vi "ziListNodesJSON.vi"(0 "Handle In":T2 {"Handle" format="0x%08x"; "Conn" format="0x%08x"}, 5 "Path (\"\")":string, 9 "Flags (None)":T3, 11 "Error In":errorcluster) -> (4 "Handle Out":T2 {"Handle" format="0x%08x"; "Conn" format="0x%08x"}, 6 "Doc":T1(array[cluster]), 15 "Error Out":errorcluster)   [LabVIEW 2018, in "Zurich Instruments LabOne.lvlib"]
doc: "Returns <b> nodes documentation </b> found at the specified path. The path may contain wild cards so that the rertuned nodes do not necessarily have to have the same parents."
uses:
  Zurich Instruments LabOne.lvlib
  <instrlib>/Zurich Instruments LabOne/Private/ziLV64.framework
  <vilib>/regexp/Match Regular Expression.xnode
  ziTypeHandle.ctl
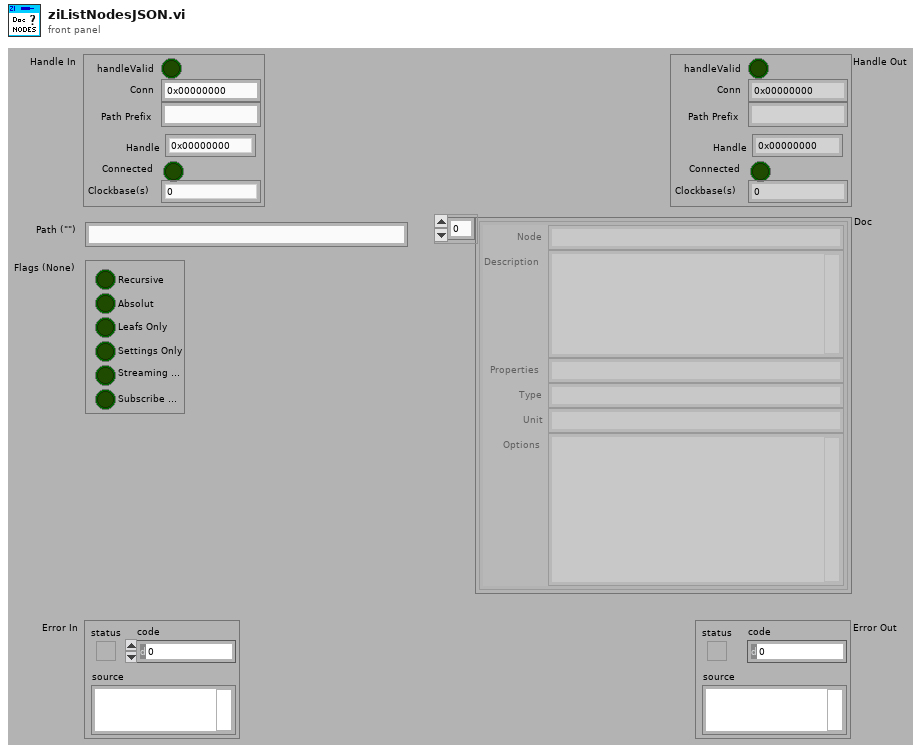
[diagram p1: front panel]
types:
  T1 = cluster{"Node":string, "Description":string, "Properties":string, "Type":string, "Unit":string, "Options":string}[]
  T2 = typedef "Zurich Instruments LabOne.lvlib/ziTypeHandle.ctl" = cluster{"handleValid":bool, "Conn":u64, "Path Prefix":string, "Handle":u64, "Connected":bool, "Clockbase(s)":dbl}
  T3 = cluster{"Recursive":bool, "Absolut":bool, "Leafs Only":bool, "Settings Only":bool, "Streaming Only":bool, "Subscribe Only":bool}
  T4 = cluster{"Node":string, "Description":string, "Properties":string, "Type":string, "Unit":string, "Options":string}
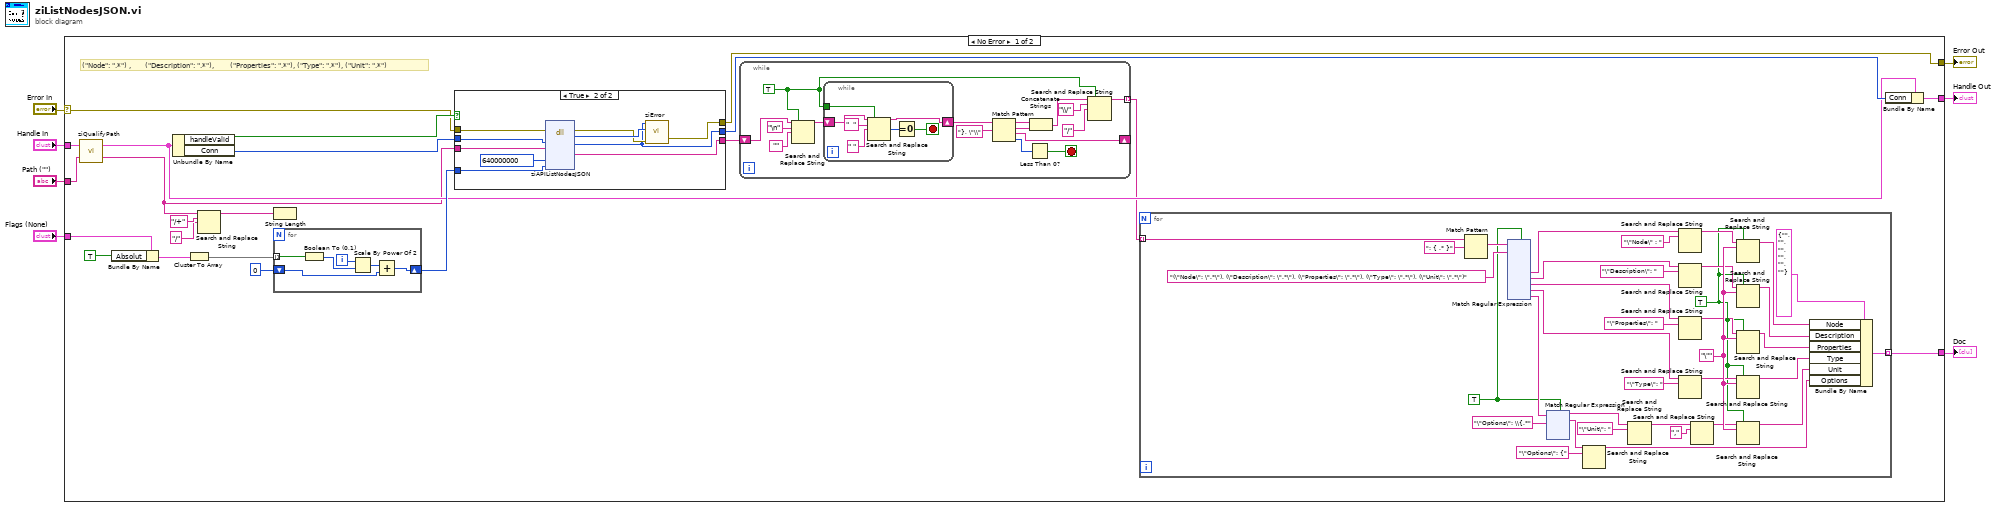
[diagram p0: block diagram]
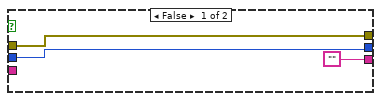
[diagram p2: hidden frame]
diagram:
  n1 = case shown="No Error" "Error In" {
    selector: "Error In" -> [w11 w329]
    tunnel: [w29 w329] -> w7
    tunnel: [w22 w328] -> w6
    tunnel: "Path (\"\")" -> [w21 _]
    tunnel: "Handle In" -> [w20 w328]
    tunnel: "Flags (None)" -> [w17 _]
    tunnel: [w9 _] -> w1
    frame No Error {
      # "(\"Node\": \".*\") ,       (\"Description\": \".*\"),        (\"Properties\": \".*\"), (\"Type\": \".*\"), (\"Unit\": \".*\")"
      n2 = call "ziQualifyPath.vi"("Path In"=w21, "Handle In"=w20) -> ("Path Out"=w12:string, "Handle Out"=w19:T2)
      n3 = Bundle By Name(cluster=w17, "Absolut"=TRUE) -> (w16:T3)
      n4 = Unbundle By Name(w19) -> ("handleValid"=w28:bool, "Conn"=w27:u64)
      n5 = Cluster To Array(cluster=w16) -> (array=w25:bool[])
      n6 = Search and Replace String(input string=w12, search string="/+" ("replace string (\"\")"), replace string="/" ("replace string (\"\")")) -> (result string=w13:string)  [unwired: 2 in, 6 out]
      n7 = String Length(string=w13) -> ()  [unwired: 1 out]
      n8 = for {
        tunnel: w25 -> [w314] mode=indexing
        shift-right: [w310] -> w23
        shift-left: 0 -> [w311]
        i -> [w309]
        n9 = Boolean To (0,1)(Boolean=w314) -> (0, 1=w313:i16)
        n10 = Scale By Power Of 2(n=w309, x=w313) -> (x*2^n=w312:i16)
        n11 = Add(x=w312, y=w311) -> (x+y=w310:i32)
      }
      n12 = case shown="True" w28 {
        tunnel: ["" w326] -> w8
        tunnel: w11 -> [w316 w324]
        tunnel: w27 -> [w315 w325]
        tunnel: [w315 w318] -> w26
        tunnel: [w316 w319] -> w29
        tunnel: w12 -> [_ w322]
        tunnel: w23 -> [_ w327]
        frame False {
        }
        frame True {
          n13 = dll-call lib="Applications/National Instruments/LabVIEW 2019 64-bit/instr.lib/Zurich Instruments LabOne/Private/ziLV*.*" fn="ziAPIListNodesJSON"(error in=w324, "Conn"=w325, "Path"=w322, "MaxLen"=640000000, "Flags"=w327) -> (error out=w320:errorcluster, "return type"=w321:u32, "Conn"=w318:u64, "Nodes"=w326:string)  [unwired: 5 in, 2 out]
          n14 = call "ziError.vi"("Conn"=w318, "ziErrorCode"=w321, "Error In"=w320) -> ("Error Out"=w319:errorcluster)  [unwired: 2 in, 1 out]
        }
      }
      n15 = while {
        shift-right: [w301] -> _
        shift-left: w8 -> [w288]
        tunnel: [w286] -> w10 mode=indexing
        stop <- w299 stop-if-true
        w289 = TRUE ("replace all? (F)")
        n16 = Search and Replace String(replace all?=w289, input string=w288, search string="\n", replace string="") -> (result string=w297:string)  [unwired: 4 in, 3 out]
        n17 = while {
          tunnel: w289 -> [w305]
          shift-right: [w304] -> w296
          shift-left: w297 -> [w308]
          stop <- w302 stop-if-true
          n18 = Search and Replace String(replace all?=w305, input string=w308, search string="  ", replace string=" " ("replace string (\"\")")) -> (result string=w304:string, number of replacements=w303:i32)  [unwired: 4 in, 2 out]
          n19 = Equal To 0?(x=w303) -> (x = 0?=w302:bool)
        }
        n20 = Match Pattern(string=w296, regular expression="}, \"\\") -> (before substring=w294:string, match substring=w295:string, after substring=w301:string, offset past match=w300:i32)  [unwired: 1 in]
        n21 = Less Than 0?(x=w300) -> (x < 0?=w299:bool)
        n22 = Concatenate Strings(w294, w295) -> (w287:string)
        n23 = Search and Replace String(replace all?=w289, input string=w287, search string="\\/", replace string="/" ("replace string (\"\")")) -> (result string=w286:string)  [unwired: 4 in, 3 out]
      }
      n24 = for {
        tunnel: w10 -> [w65] mode=indexing
        tunnel: [w42] -> w9 mode=indexing
        w30 = TRUE ("replace all? (F)")
        w39 = "\"" ("search string")
        w59 = TRUE ("multiline? (F)")
        n25 = Match Pattern(string=w65, regular expression=": { .* }") -> (match substring=w63:string)  [unwired: 1 in, 3 out]
        n26 = xnode "Match Regular Expression"("input string"=w63, "regular expression"="(\"Node\": \".*\"), (\"Description\": \".*\"), (\"Properties\": \".*\"), (\"Type\": \".*\"), (\"Unit\": \".*\")", "multiline? (F)"=w59) -> ("submatch 1"=w58:string, "submatch 2"=w57:string, "submatch 3"=w56:string, "submatch 4"=w45:string, "submatch 5"=w60:string)  [unwired: 3 in, 5 out]
        n27 = xnode "Match Regular Expression"("input string"=w60, "regular expression"="\"Options\": \\{.*", "multiline? (F)"=w59) -> ("before match"=w51:string, "whole match"=w47:string)  [unwired: 3 in, 3 out]
        n28 = Search and Replace String(input string=w47, search string="\"Options\": {" ("substring (\"\")")) -> (result string=w46:string)  [unwired: 6 in, 3 out]
        n29 = Search and Replace String(input string=w51, search string="\"Unit\": ") -> (result string=w43:string)  [unwired: 6 in, 3 out]
        n30 = Search and Replace String(input string=w58, search string="\"Node\" : ") -> (result string=w41:string)  [unwired: 6 in, 3 out]
        n31 = Search and Replace String(input string=w57, search string="\"Description\": ") -> (result string=w33:string)  [unwired: 6 in, 3 out]
        n32 = Search and Replace String(input string=w56, search string="\"Properties\": ") -> (result string=w32:string)  [unwired: 6 in, 3 out]
        n33 = Search and Replace String(input string=w45, search string="\"Type\": ") -> (result string=w31:string)  [unwired: 6 in, 3 out]
        n34 = Search and Replace String(input string=w43, search string=",") -> (result string=w38:string)  [unwired: 6 in, 3 out]
        n35 = Search and Replace String(replace all?=w30, input string=w41, search string=w39) -> (result string=w40:string)  [unwired: 5 in, 3 out]
        n36 = Search and Replace String(replace all?=w30, input string=w33, search string=w39) -> (result string=w34:string)  [unwired: 5 in, 3 out]
        n37 = Search and Replace String(replace all?=w30, input string=w32, search string=w39) -> (result string=w35:string)  [unwired: 5 in, 3 out]
        n38 = Search and Replace String(replace all?=w30, input string=w31, search string=w39) -> (result string=w36:string)  [unwired: 5 in, 3 out]
        n39 = Search and Replace String(replace all?=w30, input string=w38, search string=w39) -> (result string=w37:string)  [unwired: 5 in, 3 out]
        n40 = Bundle By Name(cluster=T4 {"Node"="", "Description"="", "Properties"="", "Type"="", "Unit"="", "Options"=""} ("output cluster 2"), "Node"=w40, "Description"=w34, "Properties"=w35, "Type"=w36, "Unit"=w37, "Options"=w46) -> (w42:T4)
      }
      n41 = Bundle By Name(cluster=w19, "Conn"=w26) -> (w22:T2)
    }
    frame Error {
    }
  }
  "Error Out" <- w7
  "Doc" <- w1
  "Handle Out" <- w6
